vi "Timestamp from String.vi"(10 "DateTime String":string, 11 "DateTimeFormatter in":refnum<class "DateTimeFormatter.lvclass">) -> (1 "Not a Timestamp?":bool, 2 "Timestamp":timestamp, 3 "DateTimeFormatter out":refnum<class "DateTimeFormatter.lvclass">)   [LabVIEW 2013, in "DateTimeFormatter.lvclass"]
uses:
  DateTimeFormatter.lvclass
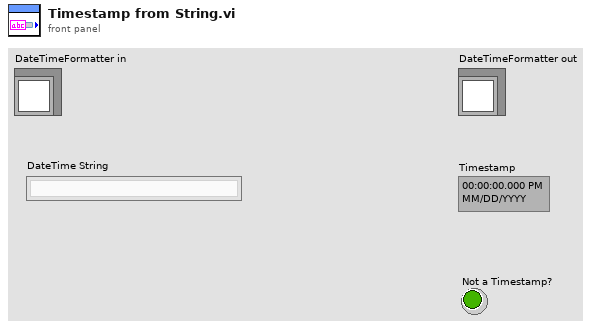
[diagram p1: front panel]
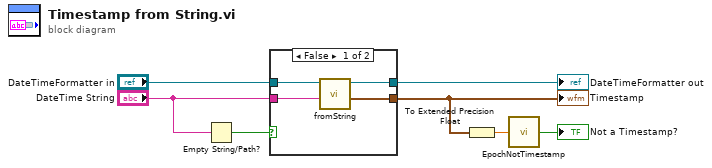
[diagram p0: block diagram]
diagram:
  n1 = Empty String/Path?(string/path="DateTime String") -> (empty?=w5:bool)
  n2 = case shown="False" w5 {
    tunnel: "DateTimeFormatter in" -> [w11 w12]
    tunnel: [w10 w12] -> w6
    tunnel: [w9 _] -> w3
    tunnel: "DateTime String" -> [w8 _]
    frame False {
      n3 = call-dynamic "fromString.vi"("DateTime String"=w8, "DateTimeFormatter in"=w11) -> ("Timestamp"=w9:timestamp, "DateTimeFormatter out"=w10:refnum<class "DateTimeFormatter.lvclass">)  [unwired: 8 in]
    }
    frame True {
    }
  }
  "DateTimeFormatter out" <- w6
  "Timestamp" <- w3
  n4 = To Extended Precision Float(1:w3) -> (0:w2:ext)
  n5 = call "EpochNotTimestamp.vi"("Epoch Time"=w2) -> ("Not a Timestamp?"=→"Not a Timestamp?":bool)  [unwired: 8 in]
